vi "Calculate-value-center.vi"(7 "Characteristics":T1[](array[typedef]), 8 "error in":errorcluster, 10 "Temp. params. ref. in":refnum<data-value>, 11 "Config. params. ref. in":refnum<data-value>) -> (0 "error IO":errorcluster, 2 "Temp. params. ref.":refnum<data-value>, 3 "Config. params. ref.":refnum<data-value>, 4 "Center index Y":i32, 6 "Center index X":i32)   [LabVIEW 2013, in "CameraVision.lvlib" / "CV-Temperature.lvclass"]
uses:
  CV-Temperature.lvclass
  Analysis/Characteristics-cluster.ctl
  Configuration/CV-Configuration.lvclass
  CV-Temperature.lvclass/CV-Temperature.ctl
  Configuration/CV-Configuration.lvclass/CV-Configuration.ctl
  Configuration/Read ROI width.vi
  Configuration/Read Width scale.vi
  Configuration/Read ROI height.vi
  Configuration/Read Height scale.vi
  Read Averaging center.vi
  Read Axis origin relative position.vi
  Read X-coordinate.vi
  Read Y-coordinate.vi
  Analysis/CV-Analysis.lvclass
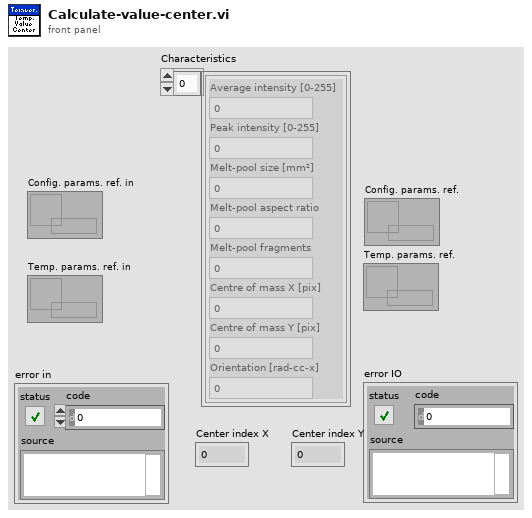
[diagram p1: front panel]
types:
  T1 = typedef "CameraVision.lvlib/CV-Analysis.lvclass/Characteristics-cluster.ctl" = cluster{"Average intensity":dbl, "Peak intensity":dbl, "Melt-pool size":dbl, "Melt-pool aspect ratio":dbl, "Melt-pool fragments":dbl, "Centre of mass X":dbl, "Centre of mass Y":dbl, "Orientation":dbl}
  T2 = enum16{"Fixed coordinates (pixel)", "Fixed coordinates (mm)", "Melt-pool center"}
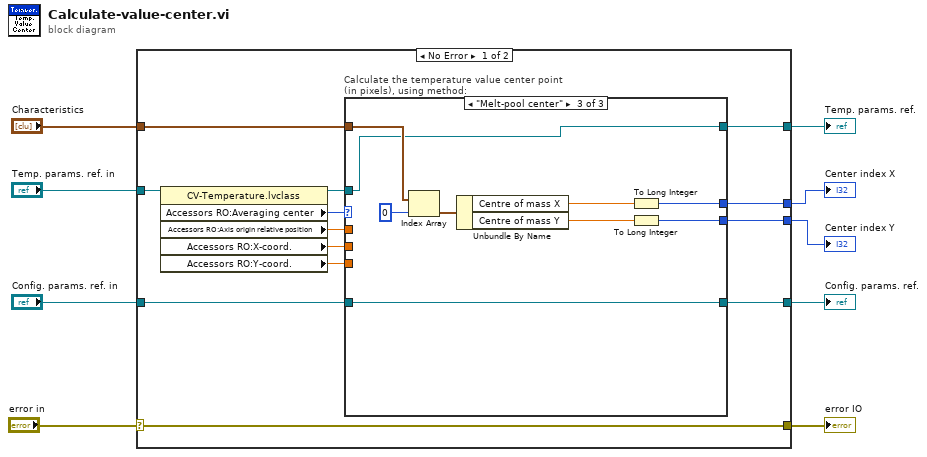
[diagram p0: block diagram]
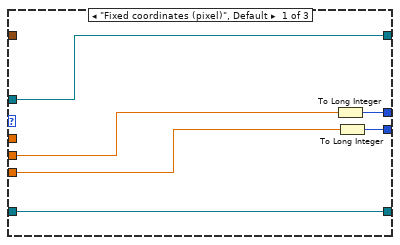
[diagram p2: hidden frame]
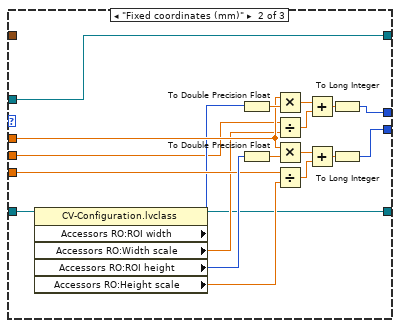
[diagram p3: hidden frame]
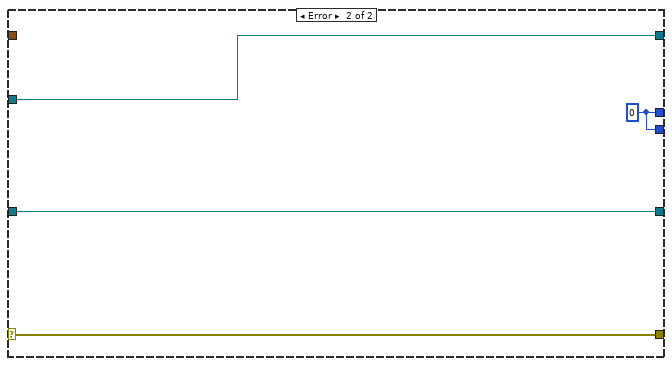
[diagram p4: hidden frame]
diagram:
  n1 = case shown="No Error" "error in" {
    selector: "error in" -> [w10 w60]
    tunnel: [w10 w60] -> w9
    tunnel: [w22 w61] -> w8
    tunnel: [w21 w61] -> w7
    tunnel: "Temp. params. ref. in" -> [w19 w59]
    tunnel: "Characteristics" -> [w20 _]
    tunnel: "Config. params. ref. in" -> [w14 w58]
    tunnel: [w13 w58] -> w2
    tunnel: [w11 w59] -> w1
    frame No Error {
      n2 = property class="CV-Temperature.lvclass"(reference=w19) -> (reference out=w12:refnum<data-value>, "Accessors RO:Averaging center"=w18:T2, "Accessors RO:Axis origin relative position"=w17:dbl, "Accessors RO:X-coord."=w16:dbl, "Accessors RO:Y-coord."=w15:dbl)  [unwired: 1 in, 1 out]
      n3 = case "Calculate the temperature value center point (in pixels), using method:" shown="\"Melt-pool center\"" w18 {
        tunnel: [w28 w40 w55] -> w21
        tunnel: [w27 w39 w53] -> w22
        tunnel: w20 -> [_ _ w51]
        tunnel: w17 -> [_ w38 _]
        tunnel: w16 -> [w26 w31 _]
        tunnel: w15 -> [w25 w34 _]
        tunnel: w14 -> [w23 w37 w49]
        tunnel: [w23 w30 w49] -> w13
        tunnel: w12 -> [w24 w29 w50]
        tunnel: [w24 w29 w50] -> w11
        frame "Fixed coordinates (pixel)", Default {
          n4 = To Long Integer(number=w26) -> (32bit integer=w28:i32)
          n5 = To Long Integer(number=w25) -> (32bit integer=w27:i32)
        }
        frame "Fixed coordinates (mm)" {
          n6 = property class="CV-Configuration.lvclass"(reference=w37) -> (reference out=w30:refnum<data-value>, "Accessors RO:ROI width"=w33:u32, "Accessors RO:Width scale"=w32:dbl, "Accessors RO:ROI height"=w35:u32, "Accessors RO:Height scale"=w36:dbl)  [unwired: 1 in, 1 out]
          n7 = To Double Precision Float(number=w33) -> (double precision float=w44:dbl)
          n8 = To Double Precision Float(number=w35) -> (double precision float=w48:dbl)
          n9 = Multiply(x=w38, y=w44) -> (x*y=w43:dbl)
          n10 = Divide(x=w31, y=w32) -> (x/y=w42:dbl)
          n11 = Multiply(x=w38, y=w48) -> (x*y=w47:dbl)
          n12 = Divide(x=w34, y=w36) -> (x/y=w46:dbl)
          n13 = Add(x=w43, y=w42) -> (x+y=w41:dbl)
          n14 = Add(x=w47, y=w46) -> (x+y=w45:dbl)
          n15 = To Long Integer(number=w41) -> (32bit integer=w40:i32)
          n16 = To Long Integer(number=w45) -> (32bit integer=w39:i32)
        }
        frame "Melt-pool center" {
          n17 = Index Array(array=w51, index=0) -> (element=w57:T1)
          n18 = Unbundle By Name(w57) -> ("Centre of mass X"=w56:dbl, "Centre of mass Y"=w54:dbl)
          n19 = To Long Integer(number=w56) -> (32bit integer=w55:i32)
          n20 = To Long Integer(number=w54) -> (32bit integer=w53:i32)
        }
      }
    }
    frame Error {
      w61 = 0
    }
  }
  "error IO" <- w9
  "Center index Y" <- w8
  "Center index X" <- w7
  "Config. params. ref." <- w2
  "Temp. params. ref." <- w1
